vi "CombineMultiTriggerSamples.vi"(8 "error in (no error)":errorcluster, 11 "SampleArraysIn":dbl[][][](array[numeric])) -> (0 "error out":errorcluster, 3 "MultiPointReadingArrayOut":T1)   [LabVIEW 2014, in "SamplerPlugins.lvlib" / "NiPxi6123.lvclass"]
uses:
  NiPxi6123.lvclass
  NISTSamplerPluginsBaseClass/TypeDefs/MultiPointReadingArrayParams.ctl
  NISTSamplerPluginsBaseClass/TypeDefs/MultiPointReadingParams.ctl
  NISTSamplerPluginsBaseClass/SamplerPluginsBase.lvclass
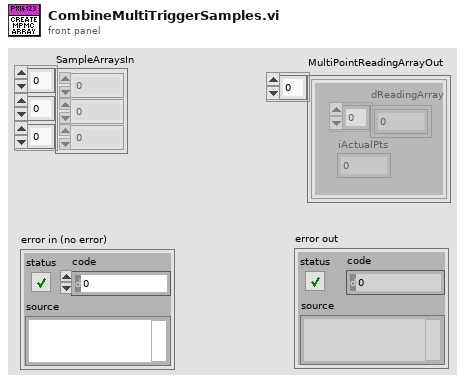
[diagram p1: front panel]
types:
  T1 = typedef "SamplerPlugins.lvlib/SamplerPluginsBase.lvclass/MultiPointReadingArrayParams.ctl" = cluster{"dReadingArray":dbl[], "iActualPts":i32}[]
  T2 = typedef "SamplerPlugins.lvlib/SamplerPluginsBase.lvclass/MultiPointReadingParams.ctl" = cluster{"dReadingArray":dbl[], "iActualPts":i32}
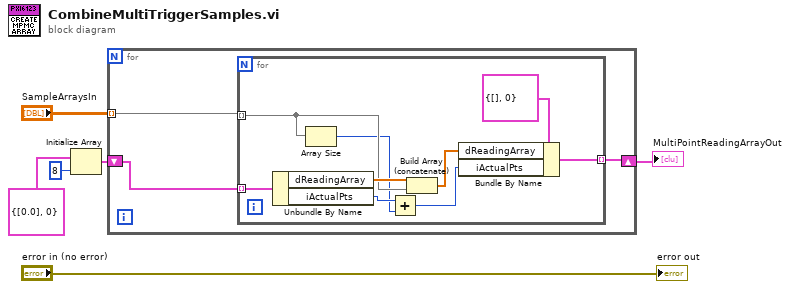
[diagram p0: block diagram]
diagram:
  n1 = Initialize Array(T2 {"dReadingArray"=[0.0], "iActualPts"=0} ("MultiPointReadingParams"), 8 ("dimension size")) -> (w1:T2[])
  n2 = for {
    tunnel: "SampleArraysIn" -> [w9] mode=indexing
    shift-right: [w8] -> w4
    shift-left: w1 -> [w7]
    n3 = for {
      tunnel: w9 -> [w16] mode=indexing
      tunnel: [w12] -> w8 mode=indexing
      tunnel: w7 -> [w18] mode=indexing
      n4 = Unbundle By Name(w18) -> ("dReadingArray"=w17:dbl[], "iActualPts"=w15:i32)
      n5 = Array Size(array=w16) -> (size(s)=w14:i32)
      n6 = Add(x=w15, y=w14) -> (x+y=w10:i32)
      n7 = Build Array (concatenate)(w17, w16) -> (w11:dbl[])
      n8 = Bundle By Name(cluster=T2 {"dReadingArray"=[], "iActualPts"=0} ("MultiPointReadingParams"), "dReadingArray"=w11, "iActualPts"=w10) -> (w12:T2)
    }
  }
  "MultiPointReadingArrayOut" <- w4
  "error out" <- "error in (no error)"
